vi "Arcade Mode.vi"(10 "Joystick In":T1 {"Right" min=-1.0 max=1.0 step=0.1 scale=-1.0..1.0; "Forward" min=-1.0 max=1.0 step=0.1 scale=-1.0..1.0}) -> (1 "Right Power":dbl(slide) scale=-1.0..1.0, 2 "Left Power":dbl(slide) scale=-1.0..1.0)   [LabVIEW 2013, in "Logical Systems.lvlib" / "Driver.lvlib"]
uses:
  Driver.lvlib
  Virtual Systems/XBox Controller/XBox Controller Class/Joystick.ctl
  XBox Controller/XBox Controller Class/Xbox Controller.lvlib
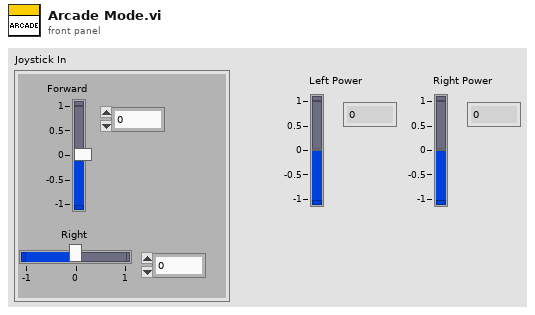
[diagram p1: front panel]
types:
  T1 = typedef "Logical Systems.lvlib/Xbox Controller.lvlib/Joystick.ctl" = cluster{"Forward":dbl, "Right":dbl}
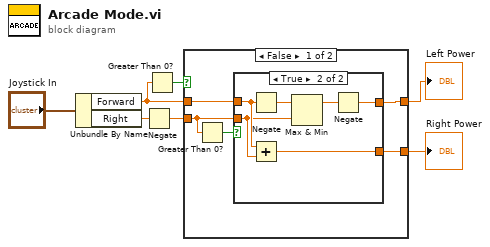
[diagram p0: block diagram]
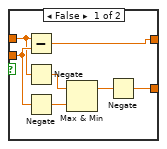
[diagram p2: hidden frame]
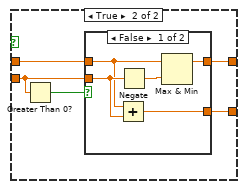
[diagram p3: hidden frame]
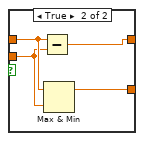
[diagram p4: hidden frame]
diagram:
  n1 = Unbundle By Name("Joystick In") -> ("Forward"=w5:dbl, "Right"=w4:dbl)
  n2 = Negate(x=w4) -> (-x=w1:dbl)
  n3 = Greater Than 0?(x=w5) -> (x > 0?=w7:bool)
  n4 = case shown="False" w7 {
    tunnel: w1 -> [w11 w29]
    tunnel: w5 -> [w10 w28]
    tunnel: [w9 w27] -> w3
    tunnel: [w8 w26] -> w2
    frame False {
      n5 = Greater Than 0?(x=w11) -> (x > 0?=w12:bool)
      n6 = case shown="True" w12 {
        tunnel: w11 -> [w19 w21]
        tunnel: w10 -> [w17 w22]
        tunnel: [w13 w23] -> w9
        tunnel: [w14 w20] -> w8
        frame False {
          n7 = Subtract(x=w17, y=w19) -> (x-y=w13:dbl)
          n8 = Negate(x=w17) -> (-x=w18:dbl)
          n9 = Negate(x=w19) -> (-x=w16:dbl)
          n10 = Max & Min(x=w18, y=w16) -> (max(x,y)=w15:dbl)  [unwired: 1 out]
          n11 = Negate(x=w15) -> (-x=w14:dbl)
        }
        frame True {
          n12 = Negate(x=w22) -> (-x=w25:dbl)
          n13 = Add(x=w22, y=w21) -> (x+y=w20:dbl)
          n14 = Max & Min(x=w25, y=w21) -> (max(x,y)=w24:dbl)  [unwired: 1 out]
          n15 = Negate(x=w24) -> (-x=w23:dbl)
        }
      }
    }
    frame True {
      n16 = Greater Than 0?(x=w29) -> (x > 0?=w30:bool)
      n17 = case shown="False" w30 {
        tunnel: w29 -> [w35 w37]
        tunnel: w28 -> [w32 w38]
        tunnel: [w33 w36] -> w27
        tunnel: [w31 w39] -> w26
        frame False {
          n18 = Add(x=w32, y=w35) -> (x+y=w31:dbl)
          n19 = Negate(x=w35) -> (-x=w34:dbl)
          n20 = Max & Min(x=w32, y=w34) -> (max(x,y)=w33:dbl)  [unwired: 1 out]
        }
        frame True {
          n21 = Subtract(x=w38, y=w37) -> (x-y=w36:dbl)
          n22 = Max & Min(x=w38, y=w37) -> (max(x,y)=w39:dbl)  [unwired: 1 out]
        }
      }
    }
  }
  "Left Power" <- w3
  "Right Power" <- w2
